vi "SPCFirstError.vi"(1 "Set/Get":bool, 2 "First Error (input)":i32=5000) -> (0 "First Error (output)":i32=5000)   [LabVIEW 2009]
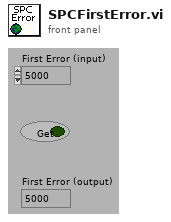
[diagram p1: front panel]
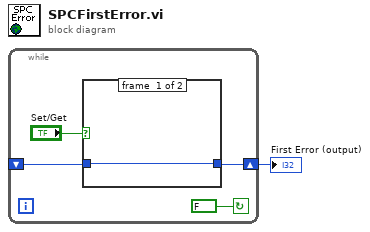
[diagram p0: block diagram]
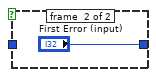
[diagram p2: hidden frame]
diagram:
  n1 = while {
    shift-right: [w3] -> w1
    shift-left: _ -> [w4]
    stop <- FALSE continue-if-true
    n2 = case shown="True" "Set/Get" {
      tunnel: [w6 "First Error (input)"] -> w3
      tunnel: w4 -> [w6 _]
      frame #0 {
      }
      frame #1 {
      }
    }
  }
  "First Error (output)" <- w1
